vi "Apply.vi"(8 "error in (no error)":errorcluster, 9 "Fs (Hz)":dbl, 10 "Array in":dbl[](array[numeric]), 11 "Gate in":refnum<class "Gate.lvclass">) -> (0 "error out":errorcluster, 2 "Array out":dbl[](array[numeric]), 3 "Gate out":refnum<class "Gate.lvclass">)   [LabVIEW 2020, in "Gate.lvclass"]
uses:
  Gate.lvclass
  Gate.lvclass/Gate.ctl
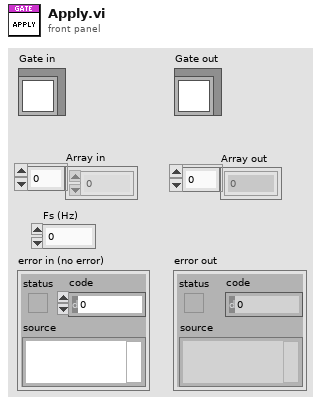
[diagram p1: front panel]
types:
  T1 = typedef "Gate.lvclass/Shape.ctl" = enum16{"OFF", "Rectangle", "Sine-squared", "Trapezoid"}
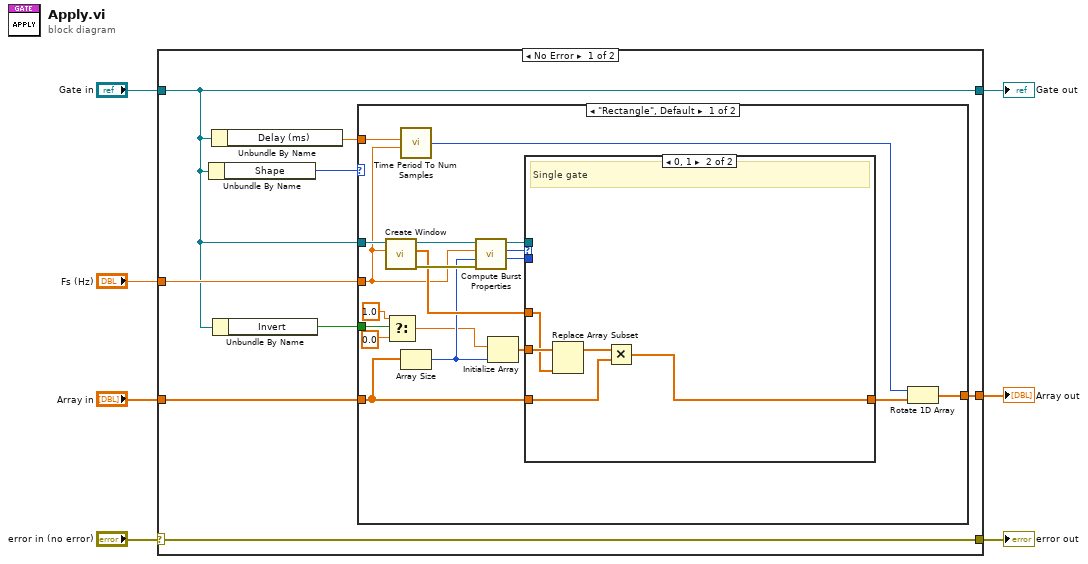
[diagram p0: block diagram]
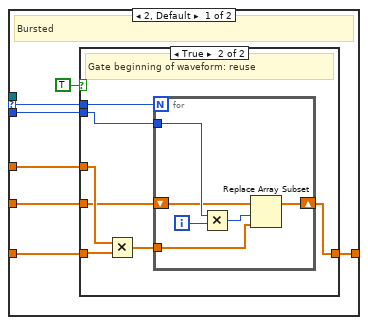
[diagram p2: hidden frame]
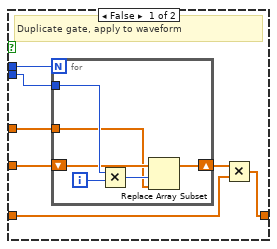
[diagram p3: hidden frame]
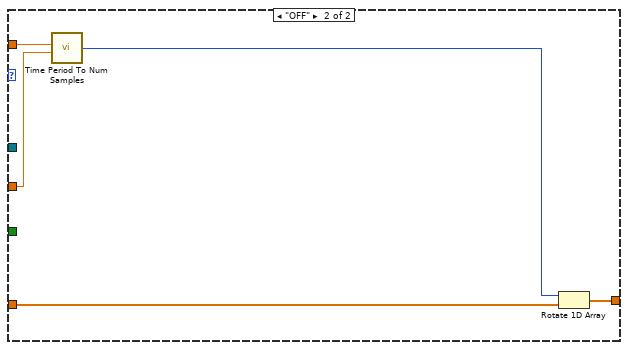
[diagram p4: hidden frame]
diagram:
  n1 = case shown="No Error" "error in (no error)" {
    selector: "error in (no error)" -> [w15 w80]
    tunnel: [w15 w80] -> w6
    tunnel: [w9 w79] -> w4
    tunnel: "Gate in" -> [w9 w79]
    tunnel: "Array in" -> [w13 w78]
    tunnel: [w12 w78] -> w2
    tunnel: "Fs (Hz)" -> [w11 _]
    frame No Error {
      n2 = Unbundle By Name(w9) -> ("Shape"=w14:T1)
      n3 = Unbundle By Name(w9) -> ("Delay (ms)"=w10:dbl)
      n4 = Unbundle By Name(w9) -> ("Invert"=w8:bool)
      n5 = case shown="\"Rectangle\", Default" w14 {
        tunnel: w13 -> [w28 w73]
        tunnel: [w23 w77] -> w12
        tunnel: w9 -> [w34 _]
        tunnel: w11 -> [w21 w75]
        tunnel: w10 -> [w22 w76]
        tunnel: w8 -> [w19 _]
        frame "Rectangle", Default {
          n6 = call "Create Window.vi"("Fs (Hz)"=w21, "Gate in"=w34) -> ("error out"=w32:errorcluster, "Window"=w29:dbl[], "Gate out"=w33:refnum<class "Gate.lvclass">)  [unwired: 7 in]
          n7 = Select(t=1.0, s=w19, f=0.0 ("element")) -> (s? t:f=w17:dbl)
          n8 = call "Time Period To Num Samples.vi"("Duration (ms)"=w22, "Sampling rate (Hz)"=w21) -> ("Samples"=w20:i32)  [unwired: 5 in]
          n9 = Array Size(array=w28) -> (size(s)=w27:i32)
          n10 = call "Compute Burst Properties.vi"("error in (no error)"=w32, "Ntotal"=w27, "Fs (Hz)"=w21, "Gate in"=w33) -> ("Points/burst cycle"=w30:i32, "#bursts"=w31:i32, "Gate out"=w25:refnum<class "Gate.lvclass">)  [unwired: 4 in, 1 out]
          n11 = Initialize Array(w17, w27) -> (w26:dbl[])
          n12 = case shown="0, 1" w31 {
            selector: w31 -> [w38 _]
            tunnel: w30 -> [w41 _]
            tunnel: w29 -> [w40 w71]
            tunnel: w28 -> [w39 w69]
            tunnel: w26 -> [w37 w72]
            tunnel: [w36 w68] -> w24
            tunnel: w25 -> [_ _]
            frame 2, Default {
              # "Bursted"
              n13 = case shown="True" TRUE {
                tunnel: w41 -> [w47 w57]
                tunnel: w40 -> [w45 w60]
                tunnel: w39 -> [w43 w61]
                tunnel: w38 -> [w48 w58]
                tunnel: w37 -> [w46 w59]
                tunnel: [w42 w55] -> w36
                frame False {
                  # "Duplicate gate, apply to waveform"
                  n14 = for {
                    N: w48 -> [_]
                    shift-right: [w50] -> w44
                    shift-left: w46 -> [w51]
                    tunnel: w47 -> [w53]
                    tunnel: w45 -> [w49]
                    i -> [w54]
                    n15 = Multiply(x=w53, y=w54) -> (x*y=w52:i32)
                    n16 = Replace Array Subset(array=w51, new element=w49, index=w52) -> (w50:dbl[])
                  }
                  n17 = Multiply(x=w44, y=w43) -> (x*y=w42:dbl[])
                }
                frame True {
                  # "Gate beginning of waveform: reuse"
                  n18 = Multiply(x=w60, y=w61) -> (x*y=w56:dbl[])
                  n19 = for {
                    N: w58 -> [_]
                    shift-right: [w62] -> w55
                    shift-left: w59 -> [w64]
                    tunnel: w57 -> [w66]
                    tunnel: w56 -> [w63]
                    i -> [w67]
                    n20 = Multiply(x=w66, y=w67) -> (x*y=w65:i32)
                    n21 = Replace Array Subset(array=w64, new element=w63, index=w65) -> (w62:dbl[])
                  }
                }
              }
            }
            frame 0, 1 {
              # "Single gate"
              n22 = Replace Array Subset(array=w72, new element=w71) -> (w70:dbl[])  [unwired: 1 in]
              n23 = Multiply(x=w70, y=w69) -> (x*y=w68:dbl[])
            }
          }
          n24 = Rotate 1D Array(1:w24, 2:w20) -> (0:w23:dbl[])
        }
        frame "OFF" {
          n25 = call "Time Period To Num Samples.vi"("Duration (ms)"=w76, "Sampling rate (Hz)"=w75) -> ("Samples"=w74:i32)  [unwired: 5 in]
          n26 = Rotate 1D Array(1:w73, 2:w74) -> (0:w77:dbl[])
        }
      }
    }
    frame Error {
    }
  }
  "error out" <- w6
  "Gate out" <- w4
  "Array out" <- w2
